vi "move_nao.vi"(3 "error in":errorcluster, 4 "node":string, 5 "Twist":T1) -> (0 "error out":errorcluster)   [LabVIEW 2015]
doc: "This VI allows the for the NAO to be moved linearly or angularly"
uses:
  ROS/Code/Console/Servers/ServerSubs/TopicDef.ctl
  ROS/Code/SubVIs/_ROSDirection.ctl
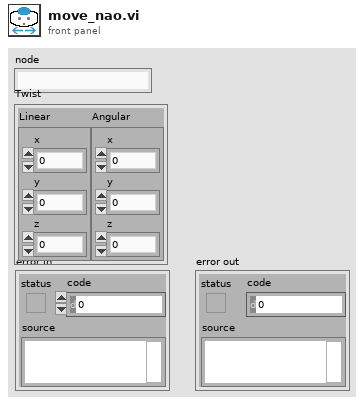
[diagram p1: front panel]
types:
  T1 = cluster{"Linear":cluster{"x":dbl, "y":dbl, "z":dbl}, "Angular":cluster{"x":dbl, "y":dbl, "z":dbl}}
  T2 = typedef "TopicDef.ctl" = cluster{"Topic":string, "Type":string, "Action":T3, "Update (ms)":u16, "queue size":u16}
  T3 = typedef "_ROSDirection.ctl" = enum16{"Node", "Publisher", "Subscriber", "ServiceClient", "ServiceProvider"}
  T4 = typedef "_ROSControl.ctl" = cluster{"topic port":u16, "Node":string, "topic":string, "type":string, "node port":u16, "error ":errorcluster, "Direction":T3, "Update (ms)":u16, "FIFO size":u16}
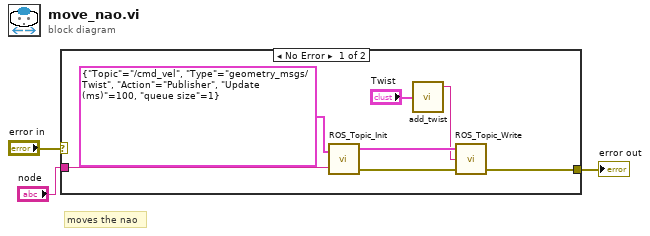
[diagram p0: block diagram]
diagram:
  # "moves the nao"
  n1 = case shown="No Error" "error in" {
    selector: "error in" -> [_ w11]
    tunnel: [w6 w11] -> w3
    tunnel: "node" -> [w8 _]
    frame No Error {
      n2 = call "ROS_Topic_Init.vi"("Definitions"=T2 {"Topic"="/cmd_vel", "Type"="geometry_msgs/Twist", "Action"=enum."Publisher", "Update (ms)"=100, "queue size"=1}, "node"=w8) -> ("ROS out"=w10:T4, "error out"=w7:errorcluster)  [unwired: 1 in]
      n3 = call "add_twist.vi"("Twist"="Twist") -> ("msg out"=w4:string)  [unwired: 4 in]
      n4 = call "ROS_Topic_Write.vi"("error in (no error)"=w7, "Msg in"=w4, "ROS in"=w10) -> ("error out"=w6:errorcluster)  [unwired: 1 in, 1 out]
    }
    frame Error {
    }
  }
  "error out" <- w3
